vi "Update Field Calibration.vi"(9 "New Field Calibration":T1 {"x locations" format="%.4g"; "coefficients" format="%.4g"}, 10 "Max Field":dbl[unit]=0.8) -> ()   [LabVIEW 2009, in "Varian Magnet.lvclass"]
doc: "GUI interface that makes sure user really wants to overwrite the Long-Term Field Calibration."
uses:
  Varian Magnet.lvclass
  <vilib>/gmath/interp.llb/in_piecewise interp poly control.ctl
  Varian Constants.vi
  Varian/Varian.lvlib
  <vilib>/gmath/NI_Gmath.lvlib
panel:
  out "Old Field\nCalibration":cluster{dbl[], dbl[]}(graph)
  out "New Field\nCalibration":cluster{dbl[], dbl[]}(graph)
  in  "Yes/No":bool
  in  "Set & Continue":bool
  # "Do you want to overwrite\nthe current long-term\ncalibration with \nthe new calibration?"
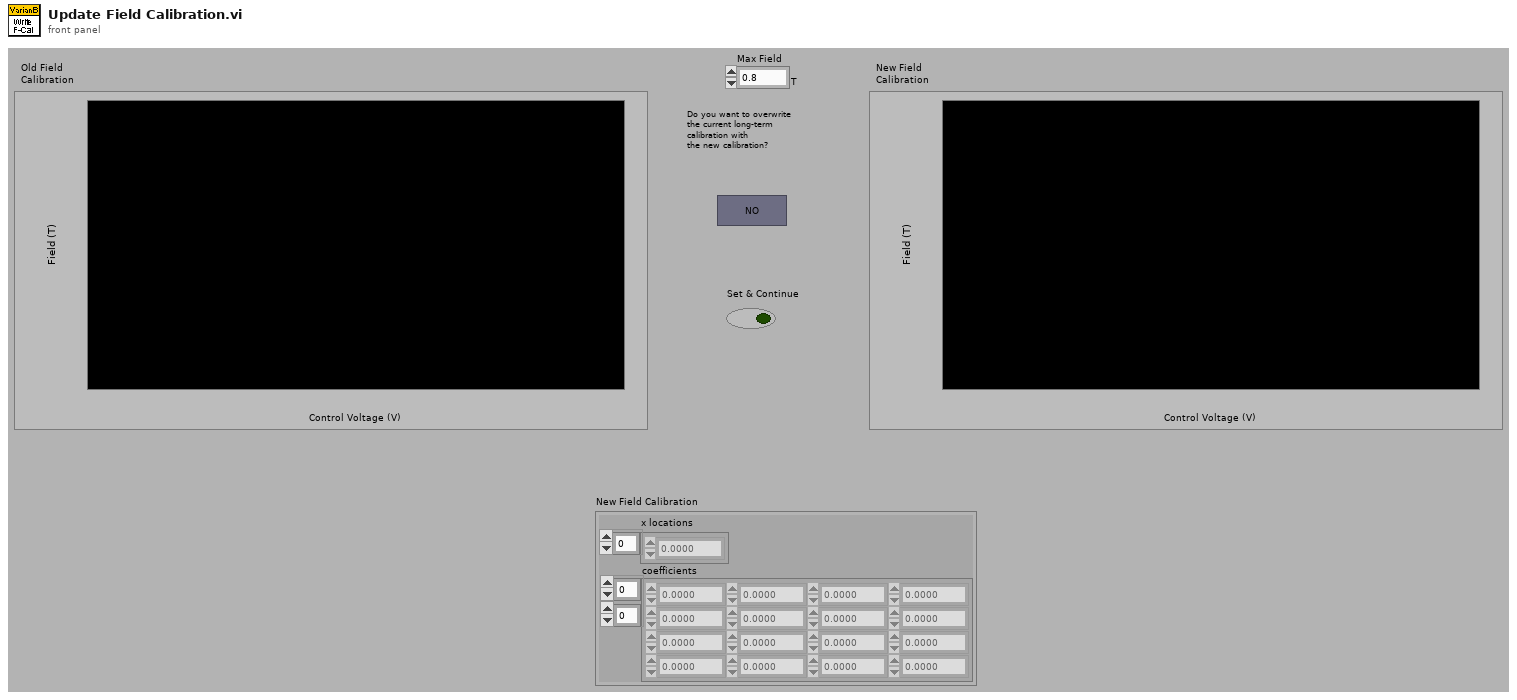
[diagram p1: front panel]
types:
  T1 = typedef "NI_Gmath.lvlib/in_piecewise interp poly control.ctl" = cluster{"x locations":dbl[], "coefficients":dbl[][]}
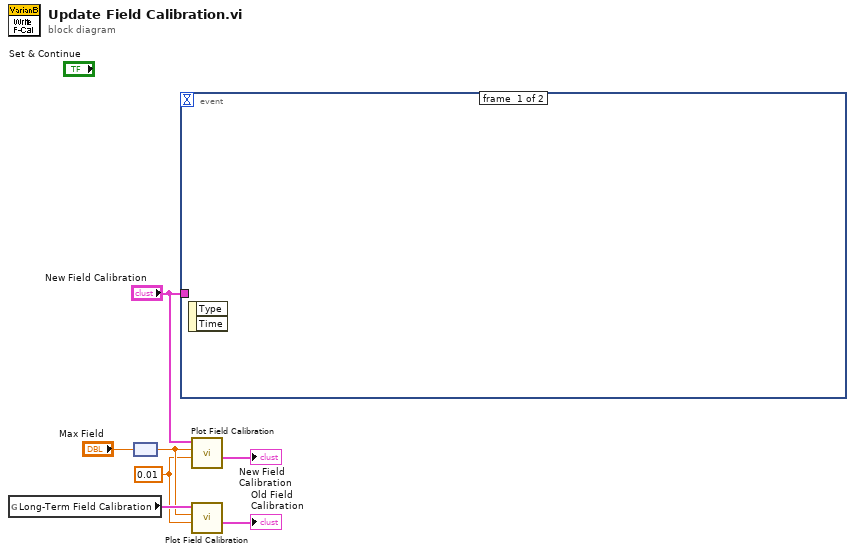
[diagram p0: block diagram]
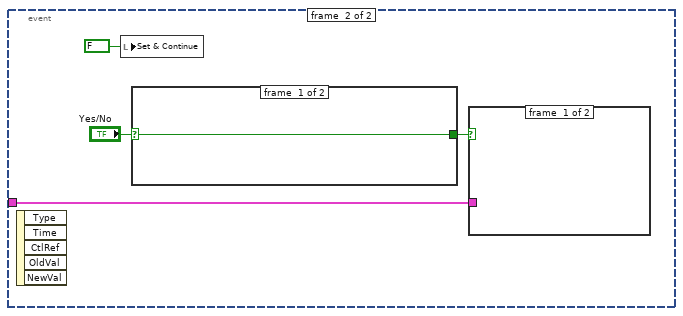
[diagram p2: hidden frame]
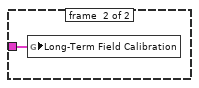
[diagram p3: hidden frame]
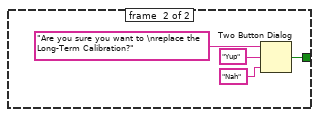
[diagram p4: hidden frame]
diagram:
  w2 = 0.01 ("x")
  n1 = global read "Varian Constants.vi" "Long-Term Field Calibration"() -> (w7:T1)
  n2 = node("Max Field") -> (w3:dbl)
  n3 = event shown="[1] \"Set & Continue\": Value Change" {
    selector: _ -> [_ _]
    dyn-events: _ -> [_ _]
    timeout: _ -> [_ _]
    tunnel: "New Field Calibration" -> [_ w9]
    event #0 {
      n4 = event-data() -> ()  [unwired: 1 in, 2 out]
    }
    event #1 {
      n5 = event-data() -> ()  [unwired: 1 in, 5 out]
      n6 = local write "Set & Continue"(FALSE) -> ()
      n7 = case shown="True" "Yes/No" {
        selector: "Yes/No" -> [w13 _]
        tunnel: [w13 w14] -> w10
        frame #0 {
        }
        frame #1 {
          n8 = Two Button Dialog(message="Are you sure you want to \nreplace the Long-Term Calibration?", 1:"Nah" ("F button name (\"Cancel\")"), 2:"Yup" ("T button name (\"OK\")")) -> (T button?=w14:bool)
        }
      }
      n9 = case shown="True" w10 {
        tunnel: w9 -> [_ w12]
        frame #0 {
        }
        frame #1 {
          n10 = global write "Varian Constants.vi" "Long-Term Field Calibration"(w12) -> ()
        }
      }
    }
  }
  n11 = call "Plot Field Calibration.vi"("Step"=w2, "Max Field"=w3, "Field Calibration"="New Field Calibration") -> ("Field Calibration Plot"=→"New Field\nCalibration":cluster{dbl[], dbl[]})  [unwired: 8 in]
  n12 = call "Plot Field Calibration.vi"("Step"=w2, "Max Field"=w3, "Field Calibration"=w7) -> ("Field Calibration Plot"=→"Old Field\nCalibration":cluster{dbl[], dbl[]})  [unwired: 8 in]
